vi "Binner - Numeric.vi"(4 "Default":dbl[][](array[numeric]), 5 "error in":errorcluster, 8 "RAW Trace":dbl[][](graph)) -> (0 "error out":errorcluster, 3 "Processed Trace":dbl[][](graph), 6 "Delay Info":T1, 7 "Spectrum Info":T2)   [LabVIEW 2013]
uses:
  controls/BinnerState.ctl
  controls/BinnerData.ctl
  <vilib>/Analysis/NI_AALBase.lvlib
panel:
  in  "Restore To Default":bool
  in  "Crop Low Bound":bool
  in  "Binned Size":u16(ring)=256 items=["64"=64, "128"=128, "256"=256, "512"=512, "1024"=1024, "2048"=2048]
  in  "Cancel":bool
  in  "OK":bool
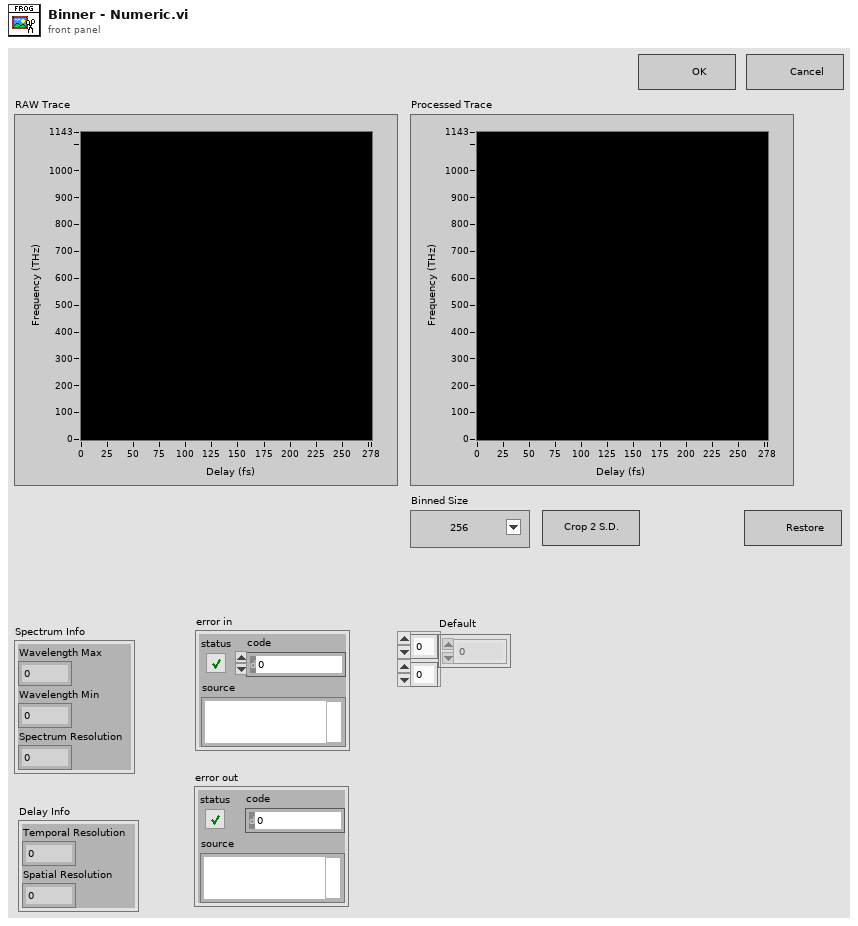
[diagram p1: front panel]
types:
  T1 = cluster{"Temporal Resolution":u16, "Spatial Resolution":u16}
  T2 = cluster{"Wavelength Max":dbl, "Wavelength Min":dbl, "Spectrum Resolution":u16}
  T3 = typedef "BinnerData.ctl" = cluster{"RAW Trace":dbl[][], "Processed Trace":dbl[][], "Spectrum Info":cluster{"Wavelength Max":dbl, "Wavelength Min":dbl, "Spectrum Resolution":u16}, "Delay Info":cluster{"Temporal Resolution":u16, "Spatial Resolution":u16}, "Binned Size":u16}
  T4 = typedef "BinnerState.ctl" = enum16{"Initialize", "Wait for Event", "Cancel", "Exit", "Binned Size", "Restore To Default", "Cursor Moved", "Crop Data", "Update Screen", "Crop 2 S.D."}
  T5 = typedef "LVRangeTypeDef.ctl" = cluster{"Minimum":dbl, "Maximum":dbl, "Increment":dbl, "Minor Increment":dbl, "Start":dbl}
  T6 = typedef "LVPointDoubleTypeDef.ctl" = cluster{"Cursor X":dbl, "Cursor Y":dbl}
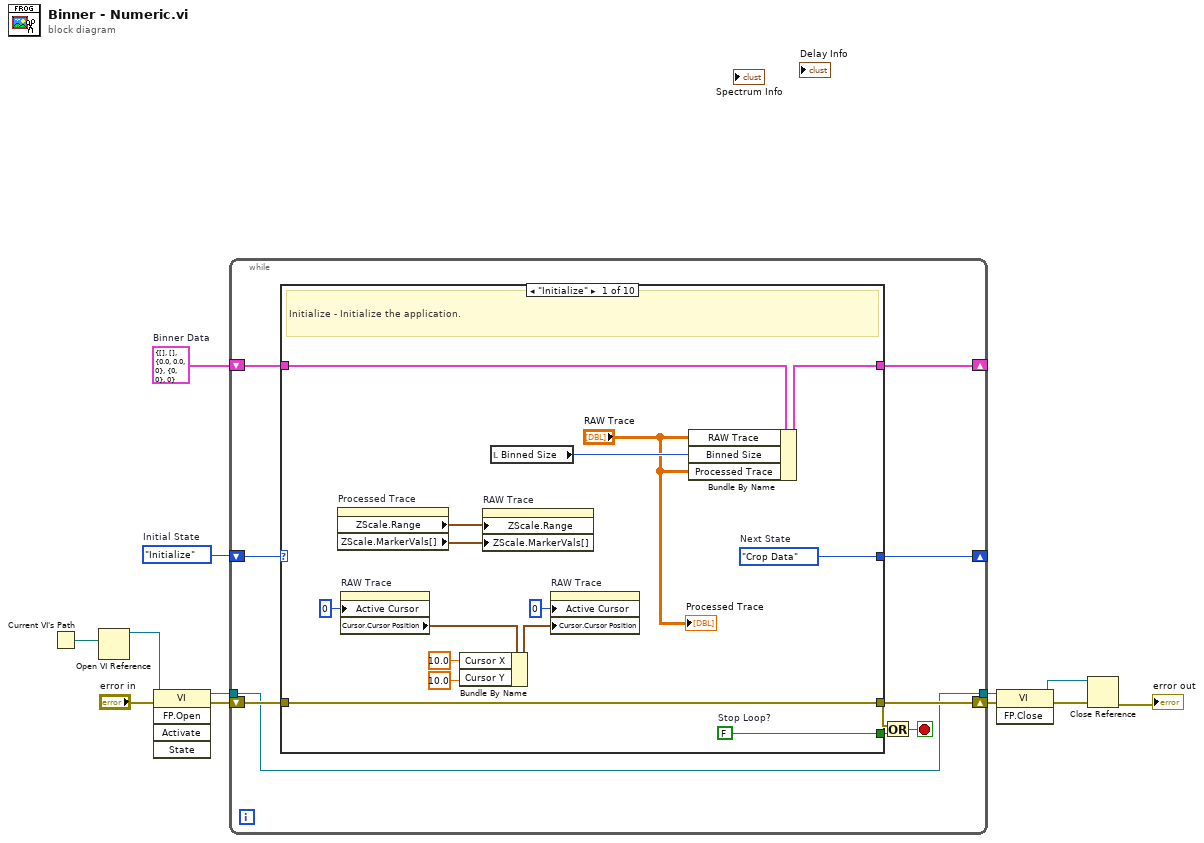
[diagram p0: block diagram]
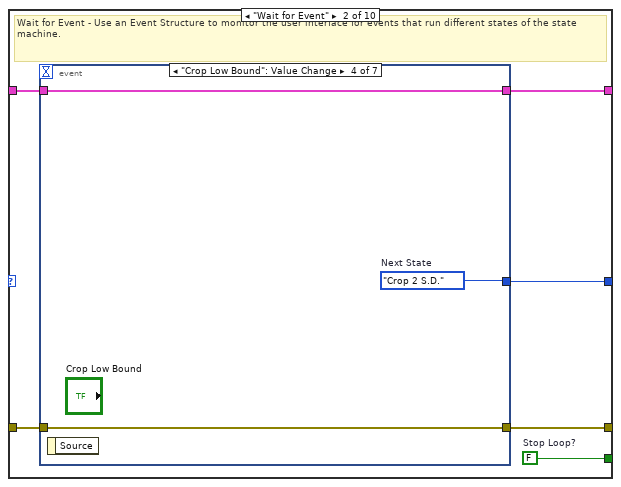
[diagram p2: hidden frame]
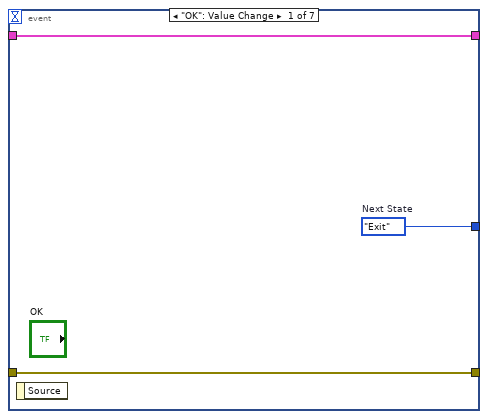
[diagram p3: hidden frame]
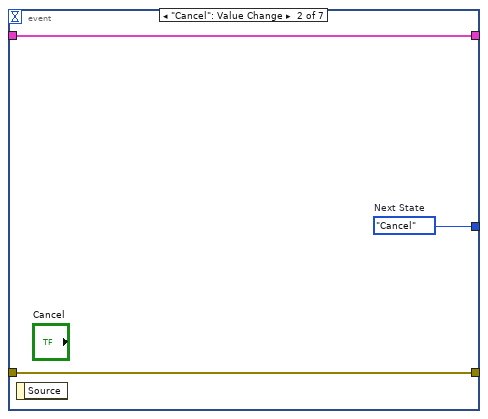
[diagram p4: hidden frame]
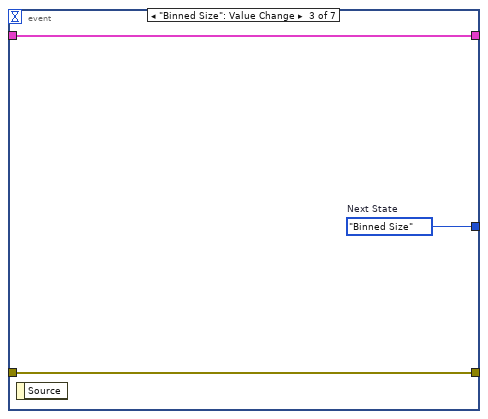
[diagram p5: hidden frame]
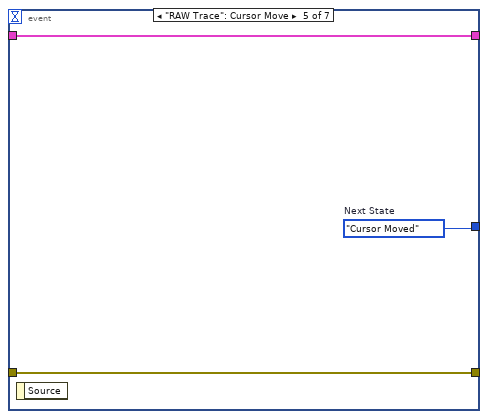
[diagram p6: hidden frame]
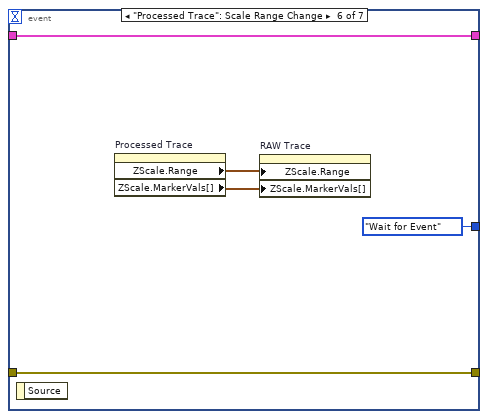
[diagram p7: hidden frame]
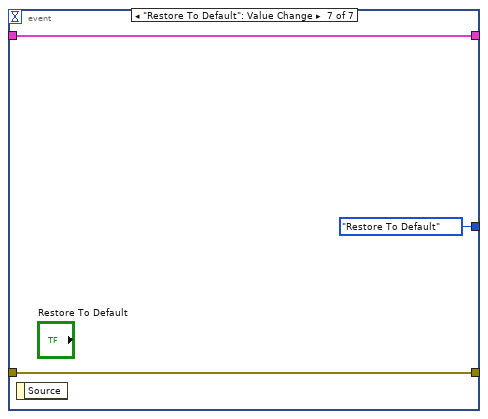
[diagram p8: hidden frame]
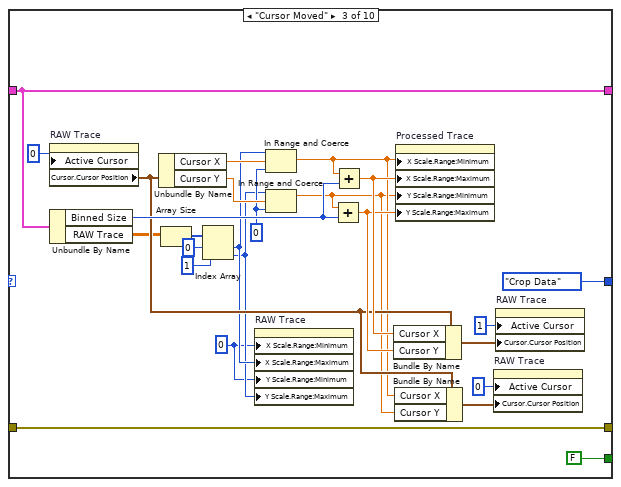
[diagram p9: hidden frame]
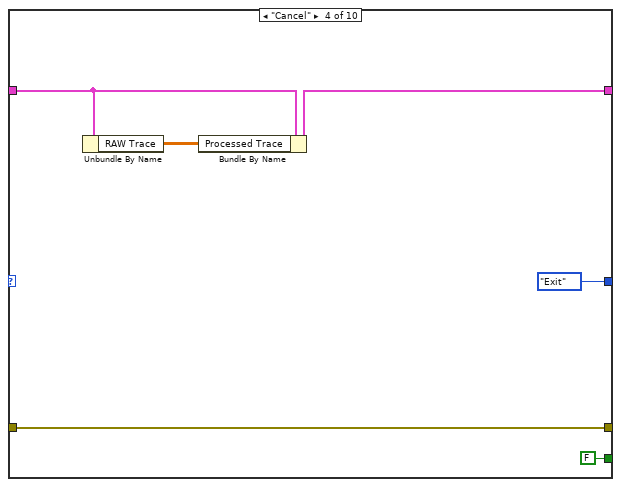
[diagram p10: hidden frame]
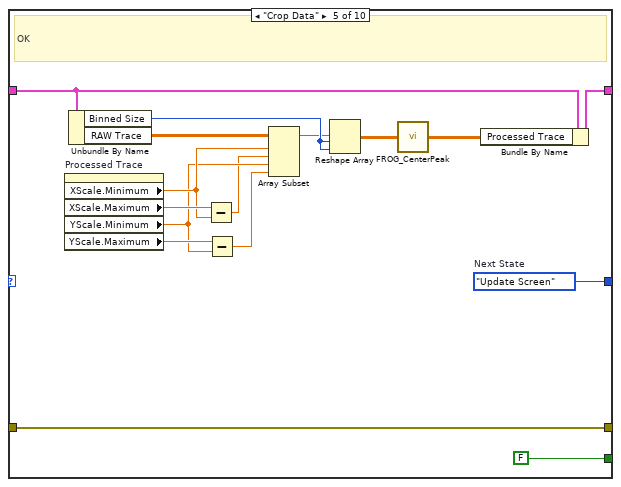
[diagram p11: hidden frame]
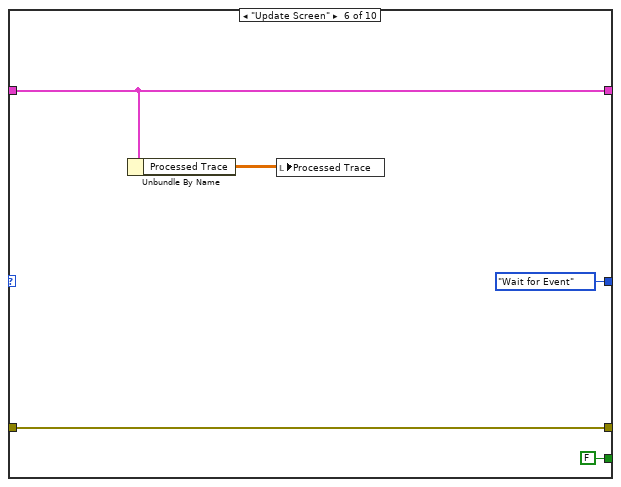
[diagram p12: hidden frame]
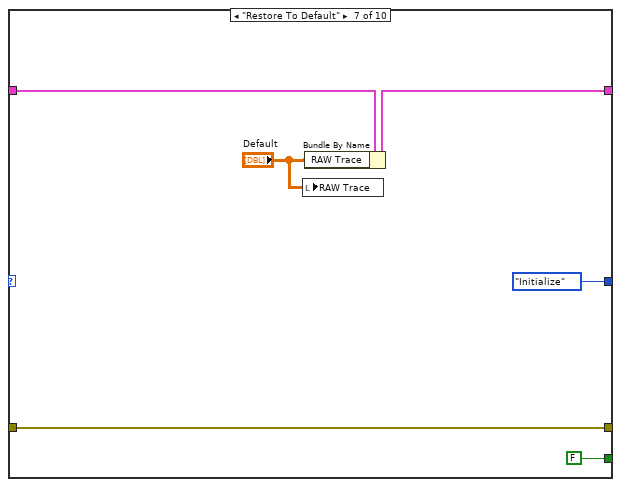
[diagram p13: hidden frame]
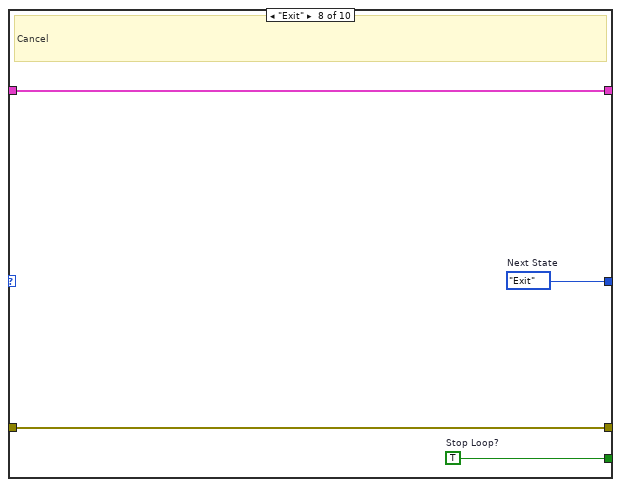
[diagram p14: hidden frame]
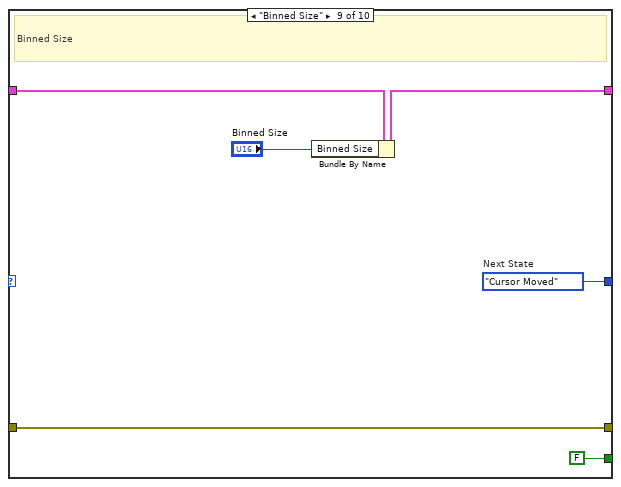
[diagram p15: hidden frame]
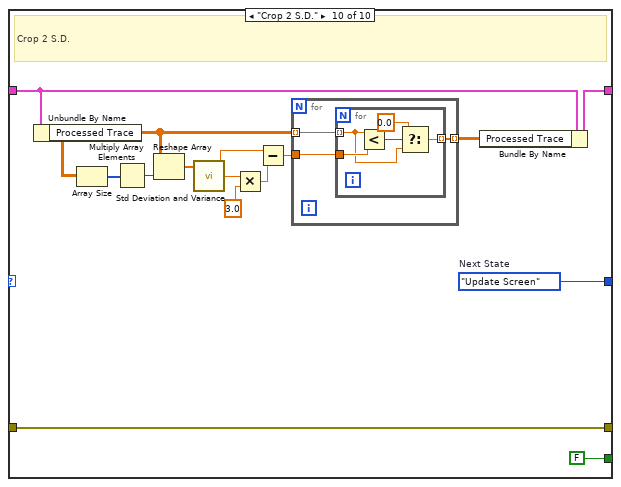
[diagram p16: hidden frame]
diagram:
  w11 = T3 {"RAW Trace"=[], "Processed Trace"=[], "Spectrum Info"={"Wavelength Max"=0.0, "Wavelength Min"=0.0, "Spectrum Resolution"=0}, "Delay Info"={"Temporal Resolution"=0, "Spatial Resolution"=0}, "Binned Size"=0}  # Binner Data
  w12 = BinnerState."Initialize"  # Initial State
  n1 = Current VI's Path() -> (path=w4:path)
  n2 = Open VI Reference(vi path=w4) -> (vi reference=w8:refnum<vi>)  [unwired: 5 in, 1 out]
  n3 = invoke class="VI" method="FP.Open"(reference=w8, error in="error in") -> (reference out=w6:refnum<vi>, error out=w9:errorcluster)  [unwired: 3 in, 3 out]
  n4 = while {
    shift-right: [w20] -> _
    shift-left: w12 -> [w21]
    shift-right: [w18] -> _
    shift-left: w11 -> [w19]
    shift-right: [w14] -> w7
    shift-left: w9 -> [w17]
    tunnel: w6 -> [w13]
    tunnel: [w13] -> w5
    stop <- w15 stop-if-true
    # "Main VI State Machine"
    n5 = case shown="\"Initialize\"" w21 {
      tunnel: [w32 w42 BinnerState."Crop Data" ("Next State") BinnerState."Exit" ("Next State") w111 BinnerState."Wait for Event" ("Next State") BinnerState."Initialize" ("Next State") w124 w131 w146] -> w20
      tunnel: [w36 w41 FALSE ("Stop Loop?") FALSE ("Stop Loop?") FALSE ("Stop Loop?") FALSE ("Stop Loop?") FALSE ("Stop Loop?") w126 FALSE ("Stop Loop?") FALSE ("Stop Loop?")] -> w16
      tunnel: w19 -> [w35 w40 w83 w93 w106 w115 w121 w127 w129 w139]
      tunnel: [w34 w39 w83 w91 w105 w115 w120 w127 w128 w138] -> w18
      tunnel: w17 -> [w33 w38 w90 w96 w110 w117 w123 w125 w133 w148]
      tunnel: [w33 w37 w90 w96 w110 w117 w123 w125 w133 w148] -> w14
      frame "Initialize" {
        w32 = BinnerState."Crop Data"  # Next State
        w36 = FALSE  # Stop Loop?
        # "Initialize - Initialize the application."
        n6 = property on="Processed Trace" class="IntGraph (strict)"() -> ("ZScale.Range"=w30:T5, "ZScale.MarkerVals[]"=w29:cluster{dbl, u32}[])  [unwired: 2 in, 2 out]
        n7 = property on="RAW Trace" class="IntGraph (strict)"("Active Cursor"=u32 0) -> ("Cursor.Cursor Position"=w25:T6)  [unwired: 2 in, 2 out]
        n8 = Bundle By Name(cluster=w25, "Cursor X"=10.0, "Cursor Y"=10.0) -> (w24:T6)
        n9 = property on="RAW Trace" class="IntGraph (strict)"("ZScale.Range"=w30, "ZScale.MarkerVals[]"=w29) -> ()  [unwired: 2 in, 2 out]
        n10 = local read "Binned Size"() -> (w31:u16)
        n11 = property on="RAW Trace" class="IntGraph (strict)"("Active Cursor"=u32 0, "Cursor.Cursor Position"=w24) -> ()  [unwired: 2 in, 2 out]
        n12 = Bundle By Name(cluster=w35, "RAW Trace"="RAW Trace", "Binned Size"=w31, "Processed Trace"="RAW Trace") -> (w34:T3)
        "Processed Trace" <- "RAW Trace"
      }
      frame "Wait for Event" {
        w41 = FALSE  # Stop Loop?
        # "Wait for Event - Use an Event Structure to monitor the user interface for events that run different states of the state machine."
        n13 = event shown="[3] \"Crop Low Bound\": Value Change" {
          selector: _ -> [_ _ _ _ _ _ _]
          dyn-events: _ -> [_ _ _ _ _ _ _]
          timeout: _ -> [_ _ _ _ _ _ _]
          tunnel: [w43 w46 w50 w52 w55 BinnerState."Wait for Event" ("Next State") BinnerState."Restore To Default" ("Next State")] -> w42
          tunnel: w40 -> [w44 w48 w49 w54 w56 w62 w63]
          tunnel: [w44 w48 w49 w54 w56 w62 w63] -> w39
          tunnel: w38 -> [w45 w47 w51 w53 w57 w61 w65]
          tunnel: [w45 w47 w51 w53 w57 w61 w65] -> w37
          event "OK": Value Change {
            w43 = BinnerState."Exit"  # Next State
            n14 = event-data() -> ()  [unwired: 1 in, 1 out]
          }
          event "Cancel": Value Change {
            w46 = BinnerState."Cancel"  # Next State
            n15 = event-data() -> ()  [unwired: 1 in, 1 out]
          }
          event "Binned Size": Value Change {
            w50 = BinnerState."Binned Size"  # Next State
            n16 = event-data() -> ()  [unwired: 1 in, 1 out]
          }
          event "Crop Low Bound": Value Change {
            w52 = BinnerState."Crop 2 S.D."  # Next State
            n17 = event-data() -> ()  [unwired: 1 in, 1 out]
          }
          event "RAW Trace": Cursor Move {
            w55 = BinnerState."Cursor Moved"  # Next State
            n18 = event-data() -> ()  [unwired: 1 in, 1 out]
          }
          event "Processed Trace": Scale Range Change {
            n19 = event-data() -> ()  [unwired: 1 in, 1 out]
            n20 = property on="Processed Trace" class="IntGraph (strict)"() -> ("ZScale.Range"=w60:T5, "ZScale.MarkerVals[]"=w59:cluster{dbl, u32}[])  [unwired: 2 in, 2 out]
            n21 = property on="RAW Trace" class="IntGraph (strict)"("ZScale.Range"=w60, "ZScale.MarkerVals[]"=w59) -> ()  [unwired: 2 in, 2 out]
          }
          event "Restore To Default": Value Change {
            n22 = event-data() -> ()  [unwired: 1 in, 1 out]
          }
        }
      }
      frame "Cursor Moved" {
        w66 = 0
        w79 = 0
        n23 = property on="RAW Trace" class="IntGraph (strict)"("Active Cursor"=u32 0) -> ("Cursor.Cursor Position"=w76:T6)  [unwired: 2 in, 2 out]
        n24 = Unbundle By Name(w83) -> ("Binned Size"=w81:u16, "RAW Trace"=w72:dbl[][])
        n25 = Unbundle By Name(w76) -> ("Cursor X"=w82:dbl, "Cursor Y"=w80:dbl)
        n26 = Array Size(array=w72) -> (size(s)=w71:i32[])
        n27 = Index Array(array=w71, index #1=0 ("index"), index #2=1 ("index")) -> (element #1=w68:i32, element #2=w67:i32)
        n28 = property on="RAW Trace" class="IntGraph (strict)"("X Scale.Range:Minimum"=w66, "X Scale.Range:Maximum"=w68, "Y Scale.Range:Minimum"=w66, "Y Scale.Range:Maximum"=w67) -> ()  [unwired: 2 in, 2 out]
        n29 = In Range and Coerce(upper limit=w68, x=w82, lower limit=w79) -> (coerced(x)=w75:dbl)  [unwired: 1 out]
        n30 = In Range and Coerce(upper limit=w67, x=w80, lower limit=w79) -> (coerced(x)=w74:dbl)  [unwired: 1 out]
        n31 = Add(x=w74, y=w81) -> (x+y=w84:dbl)
        n32 = Add(x=w75, y=w81) -> (x+y=w85:dbl)
        n33 = Bundle By Name(cluster=w76, "Cursor X"=w85, "Cursor Y"=w84) -> (w86:T6)
        n34 = Bundle By Name(cluster=w76, "Cursor X"=w75, "Cursor Y"=w74) -> (w77:T6)
        n35 = property on="Processed Trace" class="IntGraph (strict)"("X Scale.Range:Minimum"=w75, "X Scale.Range:Maximum"=w85, "Y Scale.Range:Minimum"=w74, "Y Scale.Range:Maximum"=w84) -> ()  [unwired: 2 in, 2 out]
        n36 = property on="RAW Trace" class="IntGraph (strict)"("Active Cursor"=u32 0, "Cursor.Cursor Position"=w77) -> ()  [unwired: 2 in, 2 out]
        n37 = property on="RAW Trace" class="IntGraph (strict)"("Active Cursor"=u32 1, "Cursor.Cursor Position"=w86) -> ()  [unwired: 2 in, 2 out]
      }
      frame "Cancel" {
        n38 = Unbundle By Name(w93) -> ("RAW Trace"=w92:dbl[][])
        n39 = Bundle By Name(cluster=w93, "Processed Trace"=w92) -> (w91:T3)
      }
      frame "Crop Data" {
        w111 = BinnerState."Update Screen"  # Next State
        # "OK"
        n40 = property on="Processed Trace" class="IntGraph (strict)"() -> ("XScale.Minimum"=w104:dbl, "XScale.Maximum"=w108:dbl, "YScale.Minimum"=w103:dbl, "YScale.Maximum"=w107:dbl)  [unwired: 2 in, 2 out]
        n41 = Unbundle By Name(w106) -> ("Binned Size"=w102:u16, "RAW Trace"=w109:dbl[][])
        n42 = Subtract(x=w108, y=w104) -> (x-y=w100:dbl)
        n43 = Subtract(x=w107, y=w103) -> (x-y=w101:dbl)
        n44 = Array Subset(array=w109, index (row)=w104, length (row)=w100, index (col)=w103, length (col)=w101) -> (w99:dbl[][])
        n45 = Reshape Array(w99, w102, w102) -> (w98:dbl[][])
        n46 = call "FROG_CenterPeak.vi"("Input"=w98) -> ("Output"=w97:dbl[][])
        n47 = Bundle By Name(cluster=w106, "Processed Trace"=w97) -> (w105:T3)
      }
      frame "Update Screen" {
        n48 = Unbundle By Name(w115) -> ("Processed Trace"=w114:dbl[][])
        n49 = local write "Processed Trace"(w114) -> ()
      }
      frame "Restore To Default" {
        n50 = local write "RAW Trace"("Default") -> ()
        n51 = Bundle By Name(cluster=w121, "RAW Trace"="Default") -> (w120:T3)
      }
      frame "Exit" {
        w124 = BinnerState."Exit"  # Next State
        w126 = TRUE  # Stop Loop?
        # "Cancel"
      }
      frame "Binned Size" {
        w131 = BinnerState."Cursor Moved"  # Next State
        # "Binned Size"
        n52 = Bundle By Name(cluster=w129, "Binned Size"="Binned Size") -> (w128:T3)
      }
      frame "Crop 2 S.D." {
        w146 = BinnerState."Update Screen"  # Next State
        # "Crop 2 S.D."
        n53 = Unbundle By Name(w139) -> ("Processed Trace"=w140:dbl[][])
        n54 = Array Size(array=w140) -> (size(s)=w145:i32[])
        n55 = Multiply Array Elements(1:w145) -> (0:w144:i32)
        n56 = Reshape Array(w140, w144) -> (w143:dbl[])
        n57 = call <vilib>:"Std Deviation and Variance.vi"("X"=w143) -> ("mean"=w136:dbl, "standard deviation"=w142:dbl)  [unwired: 1 in, 1 out]
        n58 = Multiply(x=w142, y=3.0) -> (x*y=w135:dbl)
        n59 = Subtract(x=w136, y=w135) -> (x-y=w134:dbl)
        n60 = for {
          tunnel: w140 -> [w151] mode=indexing
          tunnel: w134 -> [w150]
          tunnel: [w149] -> w137 mode=indexing
          n61 = for {
            tunnel: w151 -> [w153] mode=indexing
            tunnel: w150 -> [w156]
            tunnel: [w152] -> w149 mode=indexing
            n62 = Less?(x=w153, y=w156) -> (x < y?=w155:bool)
            n63 = Select(t=0.0, s=w155, f=w153) -> (s? t:f=w152:dbl)
          }
        }
        n64 = Bundle By Name(cluster=w139, "Processed Trace"=w137) -> (w138:T3)
      }
    }
    n65 = Or(x=w14, y=w16) -> (x .or. y?=w15:bool)
  }
  n66 = invoke class="VI" method="FP.Close"(reference=w5, error in=w7) -> (reference out=w1:refnum<vi>, error out=w3:errorcluster)  [unwired: 1 in, 1 out]
  n67 = Close Reference(reference=w1, error in (no error)=w3) -> (error out=→"error out":errorcluster)
